vi "WellCoordinateChecker.vi"(2 "Last Mouse Position":cluster{"X":i32, "Y":i32}, 3 "Well Coordinates":T1[](array[typedef]) {"Y" format="%.2f"; "X" format="%.2f"}) -> (0 "Well Idx":i32, 1 "Valid Point?":bool)   [LabVIEW 2022 SP3]
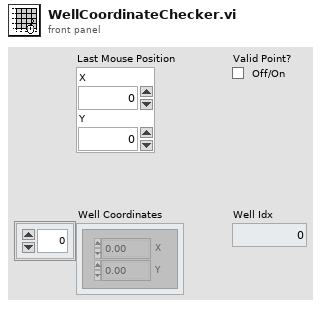
[diagram p1: front panel]
types:
  T1 = typedef "IMAQ Point" = cluster{"X":sgl, "Y":sgl}
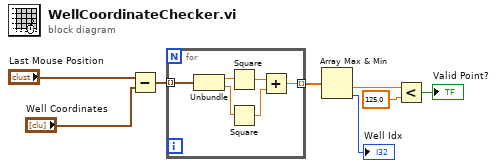
[diagram p0: block diagram]
diagram:
  n1 = Subtract(x="Last Mouse Position", y="Well Coordinates") -> (x-y=w2:T1[])
  n2 = for {
    tunnel: w2 -> [w14] mode=indexing
    tunnel: [w9] -> w3 mode=indexing
    n3 = Unbundle(w14) -> ("X"=w11:sgl, "Y"=w10:sgl)
    n4 = Square(x=w11) -> (x^2=w13:sgl)
    n5 = Square(x=w10) -> (x^2=w12:sgl)
    n6 = Add(x=w13, y=w12) -> (x+y=w9:sgl)
  }
  n7 = Array Max & Min(array=w3) -> (min value=w4:sgl, min index (indices)=→"Well Idx":i32)  [unwired: 2 out]
  n8 = Less?(x=w4, y=sgl 125.0) -> (x < y?=→"Valid Point?":bool)
